vi "Dashboard_Globals.vi"() -> ()   [LabVIEW 2018]
panel:
  in  "Mid HP Floor Arm Encoder SP":dbl
  in  "High HP Floor Arm Encoder SP":dbl
  in  "Mid HP Floor Elevator Encoder SP":dbl
  in  "High HP Floor Elevator Encoder SP":dbl
  in  "elevatorPositionActivated":bool
  in  "armPositionActivated":bool
  in  "backElevatorPositionActivated":bool
  in  "blSteerActivated":bool
  in  "brSteerActivated":bool
  in  "blDriveActivated":bool
  in  "brDriveActivated":bool
  in  "flSteerActivated":bool
  in  "frSteerActivated":bool
  in  "flDriveActivated":bool
  in  "frDriveActivated":bool
  in  "selectedAutoPlay":string
  in  "visionTargetFound":bool
  in  "emergencyDriveActivated":bool
  in  "manualElevatorActivated":bool
  in  "lastAutoPlay":string
  in  "Stow Cargo Arm Encoder SP":dbl
  in  "Depot Cargo Arm Encoder SP":dbl
  in  "Ground Cargo Arm Encoder SP":dbl
  in  "Ground HP Arm Encoder SP":dbl
  in  "Loading Station Cargo Arm Encoder SP":dbl
  in  "Loading Station HP Arm Encoder SP":dbl
  in  "Cargo Ship Cargo Arm Encoder SP":dbl
  in  "Cargo Ship HP Arm Encoder SP":dbl
  in  "Low Cargo Arm Encoder SP":dbl
  in  "Low HP Arm Encoder SP":dbl
  in  "Mid Cargo Arm Encoder SP":dbl
  in  "Mid HP Arm Encoder SP":dbl
  in  "High Cargo Arm Encoder SP":dbl
  in  "High HP Arm Encoder SP":dbl
  in  "Stow Cargo Elevator Encoder SP":dbl
  in  "Depot Cargo Elevator Encoder SP":dbl
  in  "Ground Cargo Elevator Encoder SP":dbl
  in  "Ground HP Elevator Encoder SP":dbl
  in  "Loading Station Cargo Elevator Encoder SP":dbl
  in  "Loading Station HP Elevator Encoder SP":dbl
  in  "Cargo Ship Cargo Elevator Encoder SP":dbl
  in  "Cargo Ship HP Elevator Encoder SP":dbl
  in  "Low Cargo Elevator Encoder SP":dbl
  in  "Low HP Elevator Encoder SP":dbl
  in  "Mid Cargo Elevator Encoder SP":dbl
  in  "Mid HP Elevator Encoder SP":dbl
  in  "High Cargo Elevator Encoder SP":dbl
  in  "High HP Elevator Encoder SP":dbl
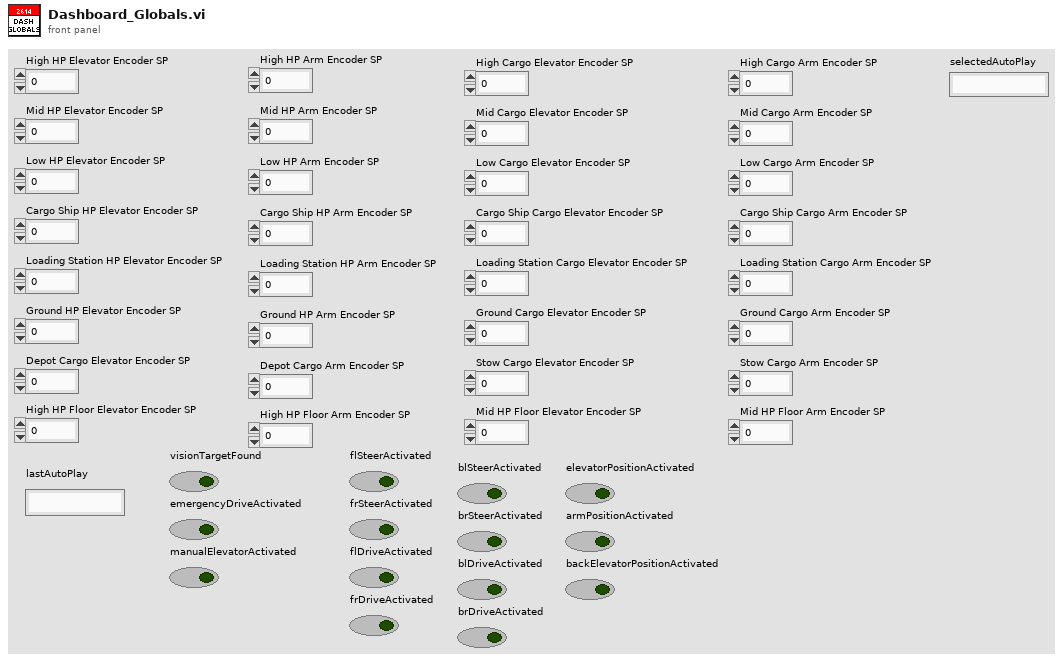
[diagram p1: front panel]
diagram:
